vi "Regelung_Abstand_.vi"() -> ()   [LabVIEW 2022 SP3]
uses:
  <vilib>/userdefined/High Color/IMAQdx.ctl
  <vilib>/Utility/file.llb/Write Delimited Spreadsheet (I64).vi
  <vilib>/Utility/file.llb/Write Delimited Spreadsheet (string).vi
  <vilib>/vision/driver/NI_Vision_Acquisition_Software.lvlib
  <vilib>/vision/NI_Vision_Development_Module.lvlib
  <vilib>/addons/control/pid/NI_PID_autopid.lvlib
panel:
  in  "Tabelle Speichern":bool
  out "Ableitung":dbl[](graph)
  out "Pixel Mittel":dbl[](graph)
  out "Distance":dbl
  in  "ROI_Int speichern":bool
  in  "ROI_Int_Aufnehmen":bool
  out "Max. Drehzahl\n(Benutzerdefinierte Einheiten)":dbl
  in  "Max. Drehzahl (U/h)":dbl=200.0
  in  "Benutzerdefinierte\nGeschwindigkeits-\neinheit":T1={"Zaehler (U)"=1.0, "Nenner (min)"=60.0, "Setzen?"=FALSE} {"Nenner (min)" format="%#_6e"}
  out "Output\nGeschwindigkeit":i32
  out "PID gains out":T2={"proportional gain (Kc)"=1.0, "integral time (Ti, min)"=0.01, "derivative time (Td, min)"=0.0} {"derivative time (Td, min)" format="%.3f"; "integral time (Ti, min)" format="%.3f"; "proportional gain (Kc)" format="%.3f"}
  in  "Autotune":bool
  in  "Startgeschwindigkeit":dbl
  in  "PID gains":T2={"proportional gain (Kc)"=1.08832, "integral time (Ti, min)"=0.041137, "derivative time (Td, min)"=0.008227} {"derivative time (Td, min)" format="%.6f"; "integral time (Ti, min)" format="%.6f"; "proportional gain (Kc)" format="%.6f"}
  in  "Sollwert":dbl
  in  "Regelung an":bool
  in  "OK Button":bool
  in  "Spacing":u8=50
  in  "n Y-Richtung":u8=3
  in  "n X-Richtung":u8=2
  in  "Größe-Radius":u8=5
  in  "Motor\nzurücksetzen":bool
  in  "Quick Stop":bool
  in  "Drehrichtung":bool
  out "Speicherpfad":string
  in  "Aufnahmen\nspeichern":bool
  in  "Speicherpfad auswählen":bool
  in  "Belichtungszeit":dbl=15000.0 min=0.0 step=500.0
  in  "Kamera":T3="cam0"
  out "ROI":T4(plugin-control)
  out "Full View":T4(plugin-control)
  out "Motordrehzahl (encoder)":i16(knob) scale=0.0..500.0
  in  "Motor Starten":bool
  in  "Motordrehzahl\nSoll":i16
  in  "VISA Motor":refnum<visa-resource-name>="COM3"
  in  "error in":errorcluster
  in  "stop":bool
  # "Motor"
  # "Kamera"
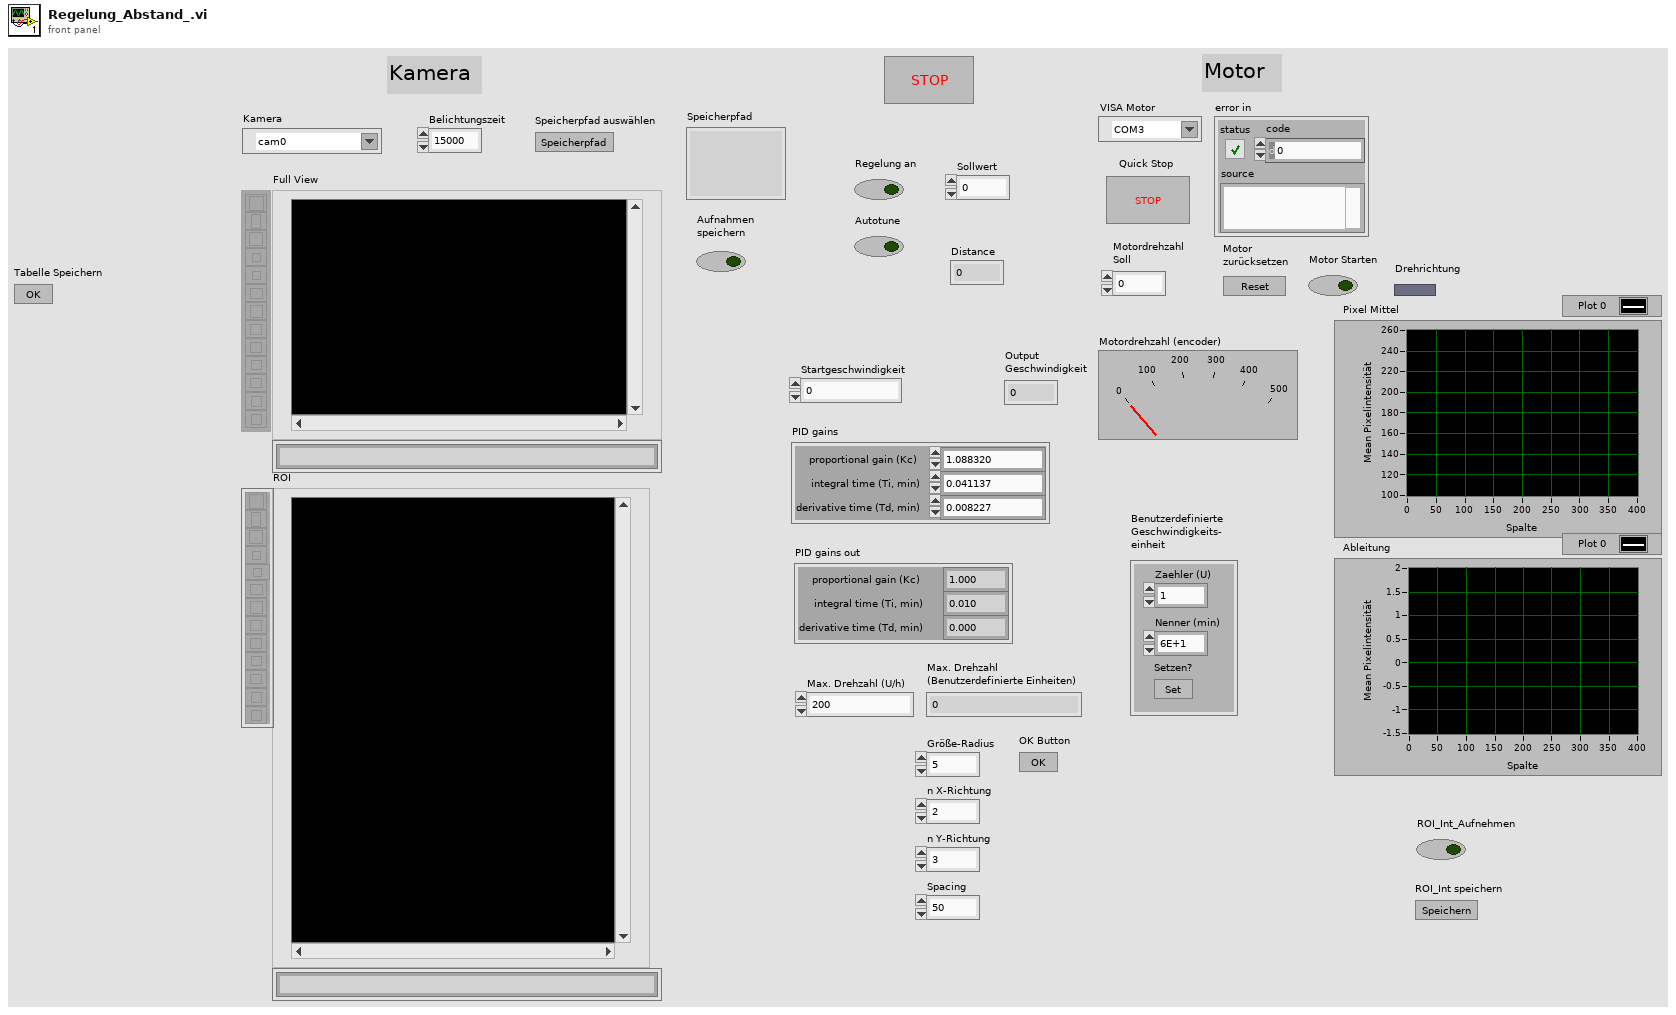
[diagram p1: front panel]
types:
  T1 = cluster{"Zaehler (U)":dbl, "Nenner (min)":dbl, "Setzen?":bool}
  T2 = cluster{"proportional gain (Kc)":dbl, "integral time (Ti, min)":dbl, "derivative time (Td, min)":dbl}
  T3 = typedef "IMAQdx.ctl" = refnum<k21>
  T4 = typedef "IMAQ Image.ctl" = refnum<image>
  T5 = typedef "Image Type" = u32
  T6 = cluster{"Data (dec)":i32, bool, "Index":string, "Sub-Index":string, "Data-Size (in Byte)":u8}
  T7 = cluster{"Index":string, "Sub-Index":string, "Data-Size (in Byte)":u8, bool}
  T8 = cluster{"Global Rectangle":i32[], "Contours":cluster{"Contour Type":u32, "ROI Type":u32, "Points":i32[]}[]}
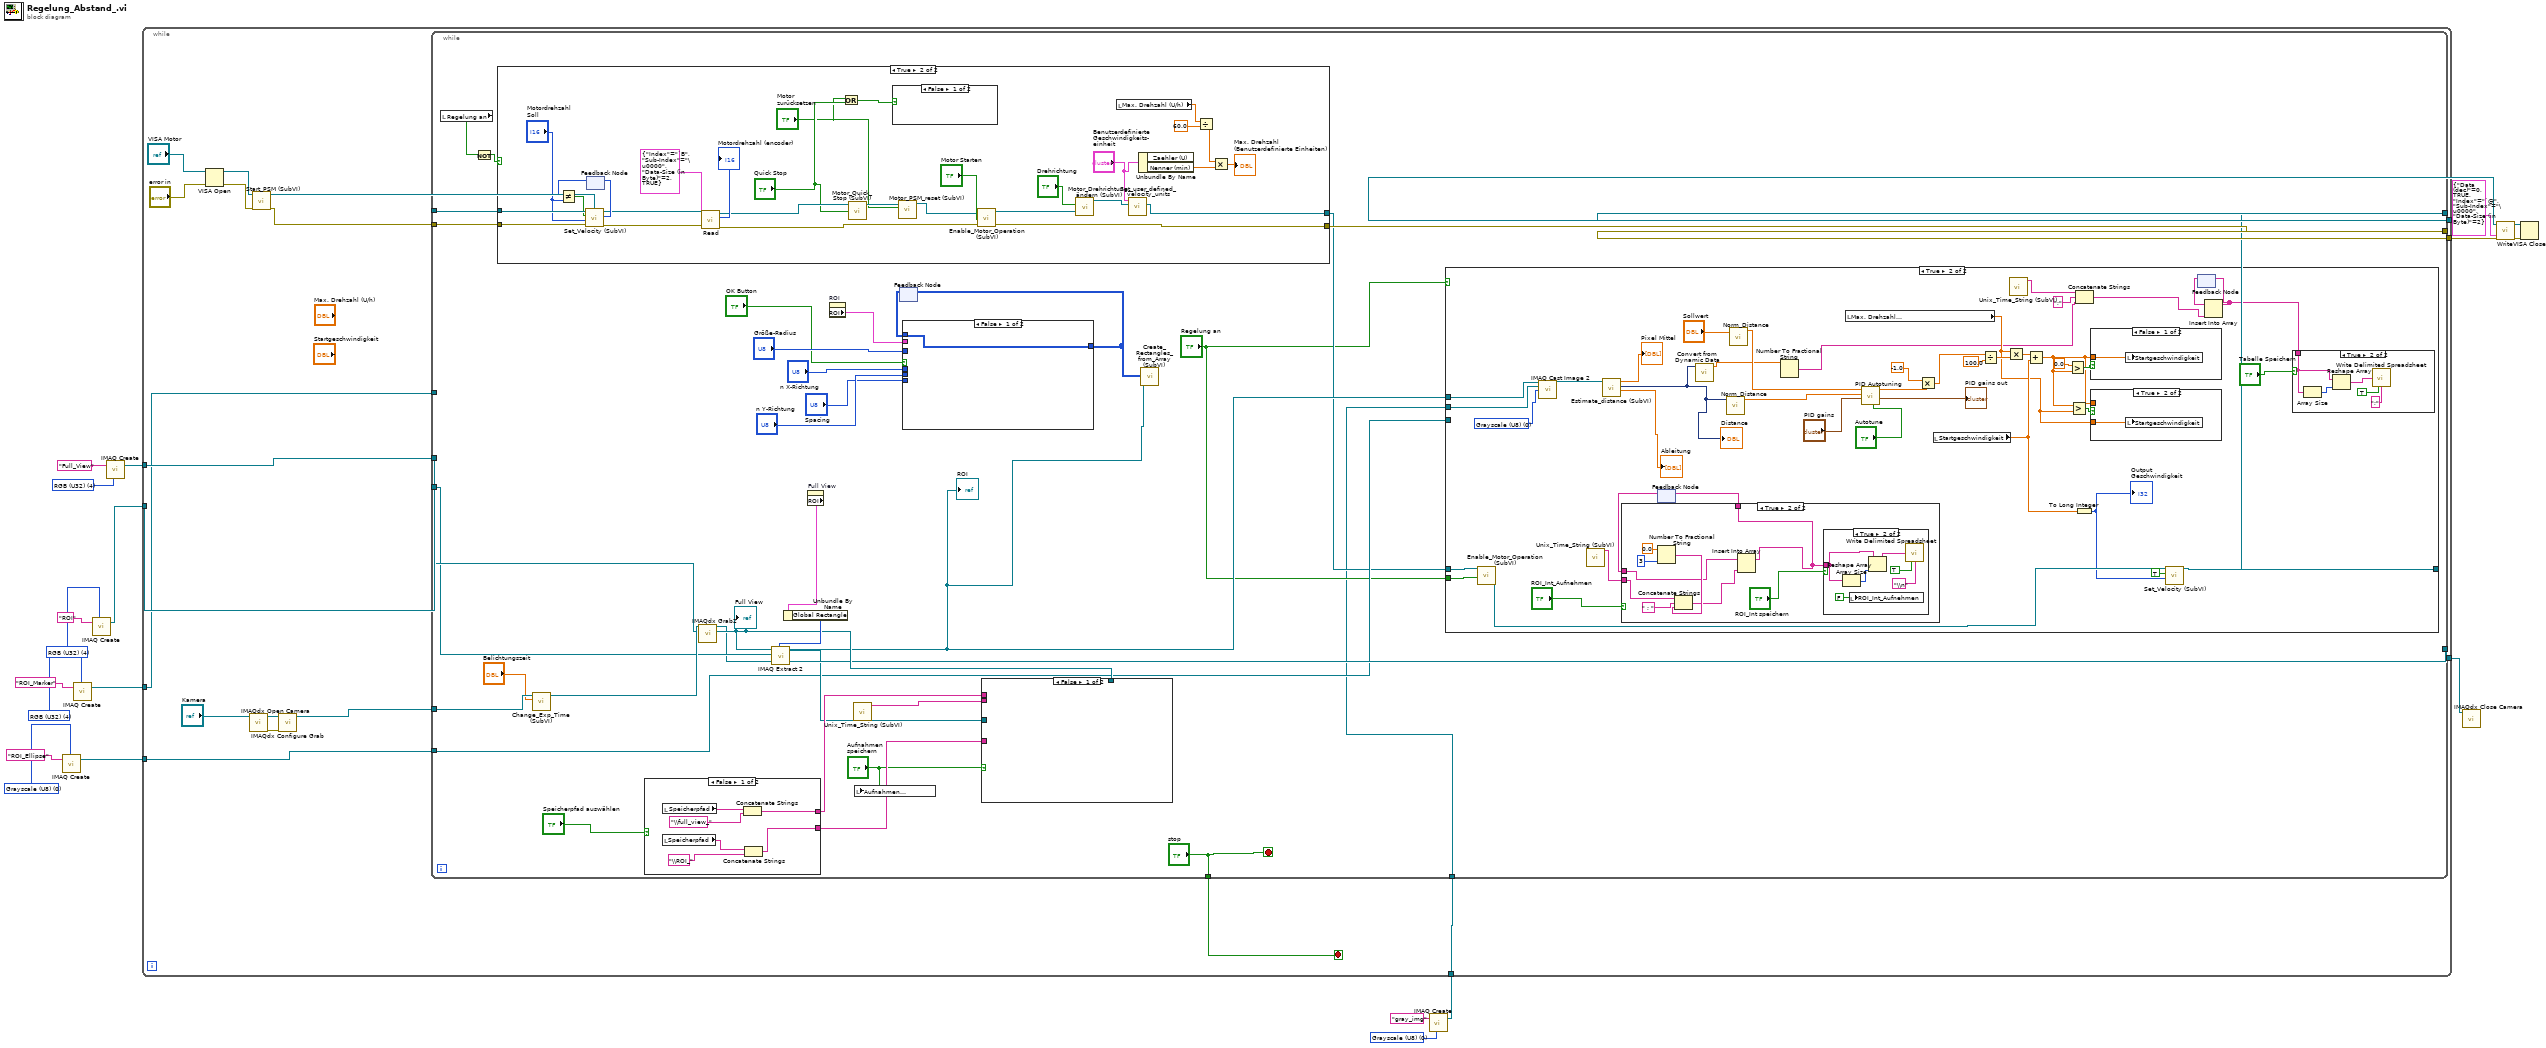
[diagram p0: block diagram]
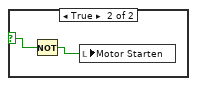
[diagram p3: hidden frame]
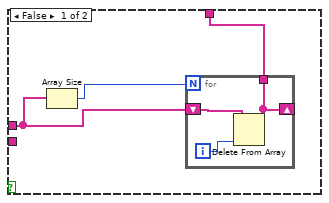
[diagram p6: hidden frame]
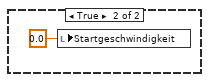
[diagram p9: hidden frame]
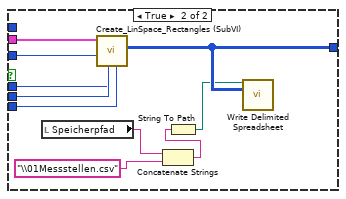
[diagram p10: hidden frame]
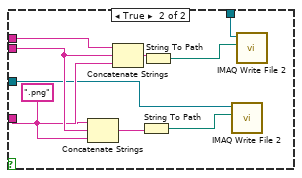
[diagram p11: hidden frame]
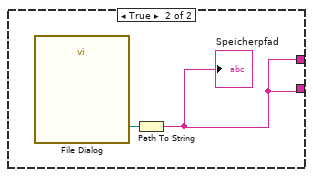
[diagram p12: hidden frame]
diagram:
  w2 = T5 0 items=["Grayscale (U8)", "Grayscale (I16)", "Grayscale (SGL)", "Complex (CSG)", "RGB (U32)", "HSL (U32)", "RGB (U64)", "Grayscale (U16)"] ("Image Type")
  w5 = T5 0 items=["Grayscale (U8)", "Grayscale (I16)", "Grayscale (SGL)", "Complex (CSG)", "RGB (U32)", "HSL (U32)", "RGB (U64)", "Grayscale (U16)"] ("Image Type")
  w8 = T5 4 items=["Grayscale (U8)", "Grayscale (I16)", "Grayscale (SGL)", "Complex (CSG)", "RGB (U32)", "HSL (U32)", "RGB (U64)", "Grayscale (U16)"] ("Image Type")
  w13 = T5 4 items=["Grayscale (U8)", "Grayscale (I16)", "Grayscale (SGL)", "Complex (CSG)", "RGB (U32)", "HSL (U32)", "RGB (U64)", "Grayscale (U16)"] ("Image Type")
  w14 = T5 4 items=["Grayscale (U8)", "Grayscale (I16)", "Grayscale (SGL)", "Complex (CSG)", "RGB (U32)", "HSL (U32)", "RGB (U64)", "Grayscale (U16)"] ("Image Type")
  n1 = call "IMAQ Create"("Image Name"="ROI_Ellipse", "Image Type"=w5) -> ("New Image"=w4:T4)  [unwired: 3 in, 1 out]
  n2 = call "IMAQ Create"("Image Name"="ROI_Marker", "Image Type"=w8) -> ("New Image"=w7:T4)  [unwired: 3 in, 1 out]
  n3 = call "IMAQ Create"("Image Name"="ROI", "Image Type"=w14) -> ("New Image"=w11:T4)  [unwired: 3 in, 1 out]
  n4 = call "IMAQ Create"("Image Name"="Full_View", "Image Type"=w13) -> ("New Image"=w12:T4)  [unwired: 3 in, 1 out]
  n5 = call "IMAQ Create"("Image Name"="gray_img", "Image Type"=w2) -> ("New Image"=w1:T4)  [unwired: 3 in, 1 out]
  n6 = while {
    tunnel: [w33] -> w18
    tunnel: [w32] -> w17
    tunnel: w12 -> [w27]
    tunnel: w11 -> [w26]
    tunnel: [w25] -> w10
    tunnel: w7 -> [w24]
    tunnel: w4 -> [w23]
    tunnel: w1 -> [w22]
    stop <- w34 stop-if-true
    n7 = VISA Open(error in (no error)="error in", VISA resource name="VISA Motor") -> (VISA resource name=w38:refnum<visa-resource-name>, error out=w37:errorcluster)  [unwired: 3 in]
    n8 = call <vilib>:"IMAQdx Open Camera.vi"("Session In"="Kamera") -> ("error out"=w30:errorcluster, "Session Out"=w29:T3)  [unwired: 9 in]
    n9 = call "Start_PSM (SubVI).vi"("error in (no error)"=w37, "VISA Refnum in"=w38) -> ("error out"=w36:errorcluster, "VISA Refnum out"=w35:refnum<visa-resource-name>)  [unwired: 8 in]
    n10 = call <vilib>:"IMAQdx Configure Grab.vi"("error in"=w30, "Session In"=w29) -> ("Session Out"=w28:T3)  [unwired: 8 in, 1 out]
    n11 = while {
      tunnel: w36 -> [w72]
      tunnel: w35 -> [w73]
      tunnel: ["stop"] -> w34
      tunnel: [w43] -> w33
      tunnel: [w71] -> w32
      tunnel: w28 -> [w70]
      tunnel: w27 -> [w68]
      tunnel: w26 -> [w65]
      tunnel: [w49] -> w25
      tunnel: w24 -> [_]
      tunnel: w23 -> [w47]
      tunnel: w22 -> [w41]
      stop <- "stop" stop-if-true
      n12 = local read "Regelung an"() -> (w46:bool)
      n13 = Not(x=w46) -> (.not. x?=w45:bool)
      n14 = case shown="True" w45 {
        tunnel: w73 -> [w76 w105]
        tunnel: w72 -> [w75 w104]
        tunnel: [w75 w98] -> w71
        tunnel: [w76 w83] -> w44
        frame False {
        }
        frame True {
          n15 = feedback #1() -> (w102:i32)  [unwired: 1 in]
          n16 = Not Equal?(x=w102, y="Motordrehzahl\nSoll") -> (x != y?=w100:bool)
          n17 = call "Set_Velocity (SubVI).vi"("error in (no error)"=w104, "Velocity in"="Motordrehzahl\nSoll", "Boolean"=w100, "VISA Refnum in"=w105) -> ("error out"=w95:errorcluster, "Velocity out"=w103:i32, "VISA Refnum out"=w97:refnum<visa-resource-name>)  [unwired: 5 in]
          n18 = feedback-in #1(w103) -> ()
          n19 = call "Read.vi"("error out"=w95, "Read"=T7 {"Index"="`B", "Sub-Index"="\u0000", "Data-Size (in Byte)"=2, TRUE}, "ComPort In"=w97) -> ("error out 2"=w94:errorcluster, "Answer"=→"Motordrehzahl (encoder)":i32, "ComPort Out"=w90:refnum<visa-resource-name>)  [unwired: 6 in]
          n20 = Or(x="Motor\nzurücksetzen", y="Quick Stop") -> (x .or. y?=w85:bool)
          n21 = call "Motor_Quick_Stop (SubVI).vi"(10:"Quick Stop", "VISA Refnum in"=w90) -> ("VISA Refnum out"=w92:refnum<visa-resource-name>)  [unwired: 9 in]
          n22 = case shown="False" w85 {
            selector: w85 -> [_ w107]
            frame False {
            }
            frame True {
              n23 = Not(x=w107) -> (.not. x?=w106:bool)
              n24 = local write "Motor Starten"(w106) -> ()
            }
          }
          n25 = call "Motor_PSM_reset (SubVI).vi"("Reset Motor"="Motor\nzurücksetzen", "VISA Refnum in"=w92) -> ("VISA Refnum out"=w91:refnum<visa-resource-name>)  [unwired: 9 in]
          n26 = call "Enable_Motor_Operation (SubVI).vi"("error in (no error)"=w94, "Motor starten in"="Motor Starten", "VISA Refnum in"=w91) -> ("error out"=w98:errorcluster, "VISA Refnum out"=w89:refnum<visa-resource-name>)  [unwired: 7 in]
          n27 = call "Motor_Drehrichtung_ändern (SubVI).vi"("Drehrichtung"="Drehrichtung", "VISA Refnum in"=w89) -> ("VISA Refnum out"=w84:refnum<visa-resource-name>)  [unwired: 9 in]
          n28 = local read "Max. Drehzahl (U/h)"() -> (w78:dbl)
          n29 = call "Set_user_defined_velocity_units.vi"("ComPort In"=w84, "Velocity user defined settings"="Benutzerdefinierte\nGeschwindigkeits-\neinheit") -> ("ComPort Out"=w83:refnum<visa-resource-name>)  [unwired: 9 in]
          n30 = Unbundle By Name("Benutzerdefinierte\nGeschwindigkeits-\neinheit") -> ("Nenner (min)"=w80:dbl)  [unwired: 1 out]
          n31 = Divide(x=w78, y=60.0) -> (x/y=w77:dbl)
          n32 = Multiply(x=w77, y=w80) -> (x*y=→"Max. Drehzahl\n(Benutzerdefinierte Einheiten)":dbl)
        }
      }
      n33 = call "Change_Exp_Time (SubVI).vi"("Belichtungszeit"="Belichtungszeit", "Refnum in"=w70) -> ("Refnum out"=w69:T3)  [unwired: 9 in]
      n34 = case shown="False" "Speicherpfad auswählen" {
        tunnel: [w202 w208] -> w50
        tunnel: [w203 w208] -> w61
        frame False {
          n35 = local read "Speicherpfad"() -> (w205:string)
          n36 = local read "Speicherpfad"() -> (w207:string)
          n37 = Concatenate Strings(w207, "\\full_view_") -> (w202:string)
          n38 = Concatenate Strings(w205, "\\ROI_") -> (w203:string)
        }
        frame True {
          n39 = call "File Dialog"() -> ("selected path"=w209:path)  [unwired: 12 in, 3 out]
          n40 = Path To String(path=w209) -> (string=w208:string)
          "Speicherpfad" <- w208
        }
      }
      n41 = call <vilib>:"IMAQdx Grab2.vi"("Image In"=w68, "Session In"=w69) -> ("Image Out"=w62:T4, "Session Out"=w49:T3)  [unwired: 6 in, 2 out]
      "Full View" <- w62
      n42 = property on="Full View" class="ImageControl"() -> ("ROI"=w67:T8)  [unwired: 2 in, 2 out]
      n43 = Unbundle By Name(w67) -> ("Global Rectangle"=w66:i32[])
      n44 = call "IMAQ Extract 2"("Optional Rectangle"=w66, "Image Dst"=w65, "Image Src"=w62) -> ("Image Dst Out"=w48:T4)  [unwired: 7 in, 1 out]
      "ROI" <- w48
      n45 = property on="ROI" class="ImageControl"() -> ("ROI"=w58:T8)  [unwired: 2 in, 2 out]
      n46 = call "Unix_Time_String (SubVI).vi"() -> ("result string"=w63:string)  [unwired: 11 in]
      n47 = local write "Aufnahmen\nspeichern"("Aufnahmen\nspeichern") -> ()
      n48 = feedback #2() -> (w52:i32[][])  [unwired: 1 in]
      n49 = case shown="False" "OK Button" {
        tunnel: w58 -> [_ w191]
        tunnel: "Größe-Radius" -> [_ w190]
        tunnel: "n Y-Richtung" -> [_ w189]
        tunnel: "n X-Richtung" -> [_ w188]
        tunnel: "Spacing" -> [_ w187]
        tunnel: [w181 w186] -> w51
        tunnel: w52 -> [w181 _]
        frame False {
        }
        frame True {
          n50 = local read "Speicherpfad"() -> (w185:string)
          n51 = call "Create_LinSpace_Rectangles (SubVI).vi"("Spacing"=w187, "n X-Richtung"=w188, "n Y-Richtung"=w189, "Größe-Radius"=w190, "ROI"=w191) -> ("output array"=w186:i32[][])  [unwired: 6 in]
          n52 = Concatenate Strings(w185, "\\01Messstellen.csv" ("string")) -> (w183:string)
          n53 = String To Path(string=w183) -> (path=w182:path)
          n54 = call-poly <vilib>:"Write Delimited Spreadsheet.vi"("file path (dialog if empty)"=w182, "2D data"=w186) -> ()  [unwired: 12 in, 2 out]
        }
      }
      n55 = feedback-in #2(w51) -> ()
      n56 = case shown="False" "Aufnahmen\nspeichern" {
        tunnel: w63 -> [_ w201]
        tunnel: w48 -> [_ w195]
        tunnel: w62 -> [_ w194]
        tunnel: w61 -> [_ w193]
        tunnel: w50 -> [_ w192]
        frame False {
        }
        frame True {
          w200 = ".png" ("string")
          n57 = Concatenate Strings(w193, w201, w200) -> (w199:string)
          n58 = Concatenate Strings(w192, w201, w200) -> (w198:string)
          n59 = String To Path(string=w199) -> (path=w196:path)
          n60 = String To Path(string=w198) -> (path=w197:path)
          n61 = call-poly "IMAQ Write File 2"("File Path"=w196, "Image"=w195) -> ()  [unwired: 8 in, 2 out]
          n62 = call-poly "IMAQ Write File 2"("File Path"=w197, "Image"=w194) -> ()  [unwired: 8 in, 2 out]
        }
      }
      n63 = call "Create_Rectangles_from_Array (SubVI).vi"("output array"=w51, "Refnum in"=w48) -> ()  [unwired: 9 in, 1 out]
      n64 = case shown="True" "Regelung an" {
        tunnel: w44 -> [w108 w145]
        tunnel: w48 -> [_ w131]
        tunnel: w47 -> [_ _]
        tunnel: [w108 w151] -> w43
        tunnel: "Regelung an" -> [_ w143]
        tunnel: w41 -> [_ w130]
        frame False {
        }
        frame True {
          w132 = T5 0 items=["Grayscale (U8)", "Grayscale (I16)", "Grayscale (SGL)", "Complex (CSG)", "RGB (U32)", "HSL (U32)", "RGB (U64)", "Grayscale (U16)"] ("Image Type")
          n65 = call "Enable_Motor_Operation (SubVI).vi"("Motor starten in"=w143, "VISA Refnum in"=w145) -> ("VISA Refnum out"=w144:refnum<visa-resource-name>)  [unwired: 8 in, 1 out]
          n66 = call "IMAQ Cast Image 2"("Image Src"=w131, "Image Dst"=w130, "Image Type"=w132) -> ("Image Dst Out"=w121:T4)  [unwired: 11 in, 1 out]
          n67 = call "Unix_Time_String (SubVI).vi"() -> ("result string"=w136:string)  [unwired: 11 in]
          n68 = call "Estimate_distance (SubVI).vi"("Refnum in"=w121) -> ("Waveform Graph 2"=→"Ableitung":dbl[], "Dynamic Data"=w115:dynamicdata, "Waveform Graph"=→"Pixel Mittel":dbl[])  [unwired: 8 in]
          "Distance" <- w115
          n69 = feedback #3() -> (w134:string[])  [unwired: 1 in]
          n70 = case shown="True" "ROI_Int_Aufnehmen" {
            tunnel: w136 -> [_ w171]
            tunnel: [w159 w165] -> w133
            tunnel: w134 -> [w157 w164]
            frame False {
              n71 = Array Size(array=w157) -> (size(s)=w158:i32)
              n72 = for {
                N: w158 -> [_]
                tunnel: [w161] -> w159
                shift-right: [w161] -> _
                shift-left: w157 -> [w162]
                i -> [w160]
                n73 = Delete From Array(array=w162, index=w160) -> (array with subset deleted=w161:string[])  [unwired: 1 in, 1 out]
              }
            }
            frame True {
              n74 = Number To Fractional String(number=0.0, precision (6)=i16 3) -> (F-format string=w168:string)  [unwired: 2 in]
              n75 = Concatenate Strings(w171, " ; " ("string"), w168) -> (w166:string)
              n76 = Insert Into Array(array=w164, new element=w166) -> (w165:string[])  [unwired: 1 in]
              n77 = case shown="True" "ROI_Int speichern" {
                tunnel: w165 -> [_ w176]
                frame False {
                }
                frame True {
                  n78 = Array Size(array=w176) -> (size(s)=w174:i32)
                  n79 = local write "ROI_Int_Aufnehmen"(FALSE ("ROI_Int_Aufnehmen")) -> ()
                  n80 = Reshape Array(w176, w174) -> (w175:string[])
                  n81 = call-poly <vilib>:"Write Delimited Spreadsheet.vi"("1D data"=w175, "transpose? (no:F)"=TRUE, "delimiter (\\t)"="\\n" ("delimiter (\\t)")) -> ()  [unwired: 11 in, 2 out]
                }
              }
            }
          }
          n82 = feedback-in #3(w133) -> ()
          n83 = call "Convert from Dynamic Data"("Dynamic Data Type"=w115) -> ("Array"=w110:dbl[])  [unwired: 3 in]
          n84 = call "Norm_Distance.vi"("Distance"=w115) -> ("Numeric"=w124:sgl)  [unwired: 10 in]
          n85 = call "Norm_Distance.vi"("Distance"="Sollwert") -> ("Numeric"=w125:sgl)  [unwired: 10 in]
          n86 = Number To Fractional String(number=w110) -> (F-format string=w109:string[])  [unwired: 3 in]
          n87 = local read "Max. Drehzahl\n(Benutzerdefinierte Einheiten)"() -> (w137:dbl)
          n88 = call <vilib>:"PID Autotuning.vi"("autotune? (F)"="Autotune", "PID gains"="PID gains", "process variable"=w124, "setpoint"=w125) -> ("PID gains out"=→"PID gains out":T2, "output"=w126:dbl)  [unwired: 4 in, 2 out]
          n89 = Multiply(x=-1.0, y=w126) -> (x*y=w128:dbl)
          n90 = local read "Startgeschwindigkeit"() -> (w142:dbl)
          n91 = Divide(x=w128, y=100.0) -> (x/y=w139:dbl)
          n92 = Multiply(x=w137, y=w139) -> (x*y=w150:dbl)
          n93 = call "Unix_Time_String (SubVI).vi"() -> ("result string"=w116:string)  [unwired: 11 in]
          n94 = Add(x=w150, y=w142) -> (x+y=w141:dbl)
          n95 = Greater?(x=0.0, y=w141) -> (0:w146:bool)
          n96 = Greater?(x=w141, y=w137) -> (0:w148:bool)
          n97 = To Long Integer(number=w142) -> (32bit integer=w140:i32)
          "Output\nGeschwindigkeit" <- w140
          n98 = Concatenate Strings(w116, ";" ("string"), w109) -> (w112:string)
          n99 = case shown="False" w146 {
            tunnel: w141 -> [w179 _]
            frame False {
              n100 = local write "Startgeschwindigkeit"(w179) -> ()
            }
            frame True {
              n101 = local write "Startgeschwindigkeit"(0.0 ("Startgeschwindigkeit")) -> ()
            }
          }
          n102 = case shown="True" w148 {
            tunnel: w141 -> [_ _]
            tunnel: w137 -> [_ w178]
            frame False {
            }
            frame True {
              n103 = local write "Startgeschwindigkeit"(w178) -> ()
            }
          }
          n104 = call "Set_Velocity (SubVI).vi"("Velocity in"=w140, "Boolean"=TRUE, "VISA Refnum in"=w144) -> ("VISA Refnum out"=w151:refnum<visa-resource-name>)  [unwired: 6 in, 2 out]
          n105 = feedback #4() -> (w111:string[])  [unwired: 1 in]
          n106 = Insert Into Array(array=w111, new element=w112) -> (w113:string[])  [unwired: 1 in]
          n107 = feedback-in #4(w113) -> ()
          n108 = case shown="True" "Tabelle Speichern" {
            tunnel: w113 -> [_ w156]
            frame False {
            }
            frame True {
              n109 = Array Size(array=w156) -> (size(s)=w155:i32)
              n110 = Reshape Array(w156, w155) -> (w154:string[])
              n111 = call-poly <vilib>:"Write Delimited Spreadsheet.vi"("1D data"=w154, "transpose? (no:F)"=TRUE, "delimiter (\\t)"=";" ("delimiter (\\t)")) -> ()  [unwired: 11 in, 2 out]
            }
          }
        }
      }
    }
  }
  n112 = call <vilib>:"IMAQdx Close Camera.vi"("Session In"=w10) -> ()  [unwired: 10 in, 1 out]
  n113 = call "Write.vi"("error in"=w17, "Write"=T6 {"Data (dec)"=0, TRUE, "Index"="`@", "Sub-Index"="\u0000", "Data-Size (in Byte)"=2}, "ComPort In"=w18) -> ("error out"=w19:errorcluster, "ComPort Out"=w20:refnum<visa-resource-name>)  [unwired: 7 in]
  n114 = VISA Close(VISA resource name=w20, error in (no error)=w19) -> ()  [unwired: 1 out]
